vi "Simple_DAQ_PressureTime_Graph.vi"() -> ()   [LabVIEW 2021]
panel:
  in  "See Log FilePath":bool
  out "Log File Name":string
  out "Log Date & Time":string
  out "Log File Path":path
  out "error out":errorcluster
  in  "Start Logging":bool
  out "Pressure Chart":dbl[](graph)
  out "Date & Time":string
  out "Pressure (Bar)":dbl format="%#2_4f"
  in  "Start Aquisition":bool
  out "Voltage Detected":dbl format="%0.2f"
  in  "Stop Button":bool
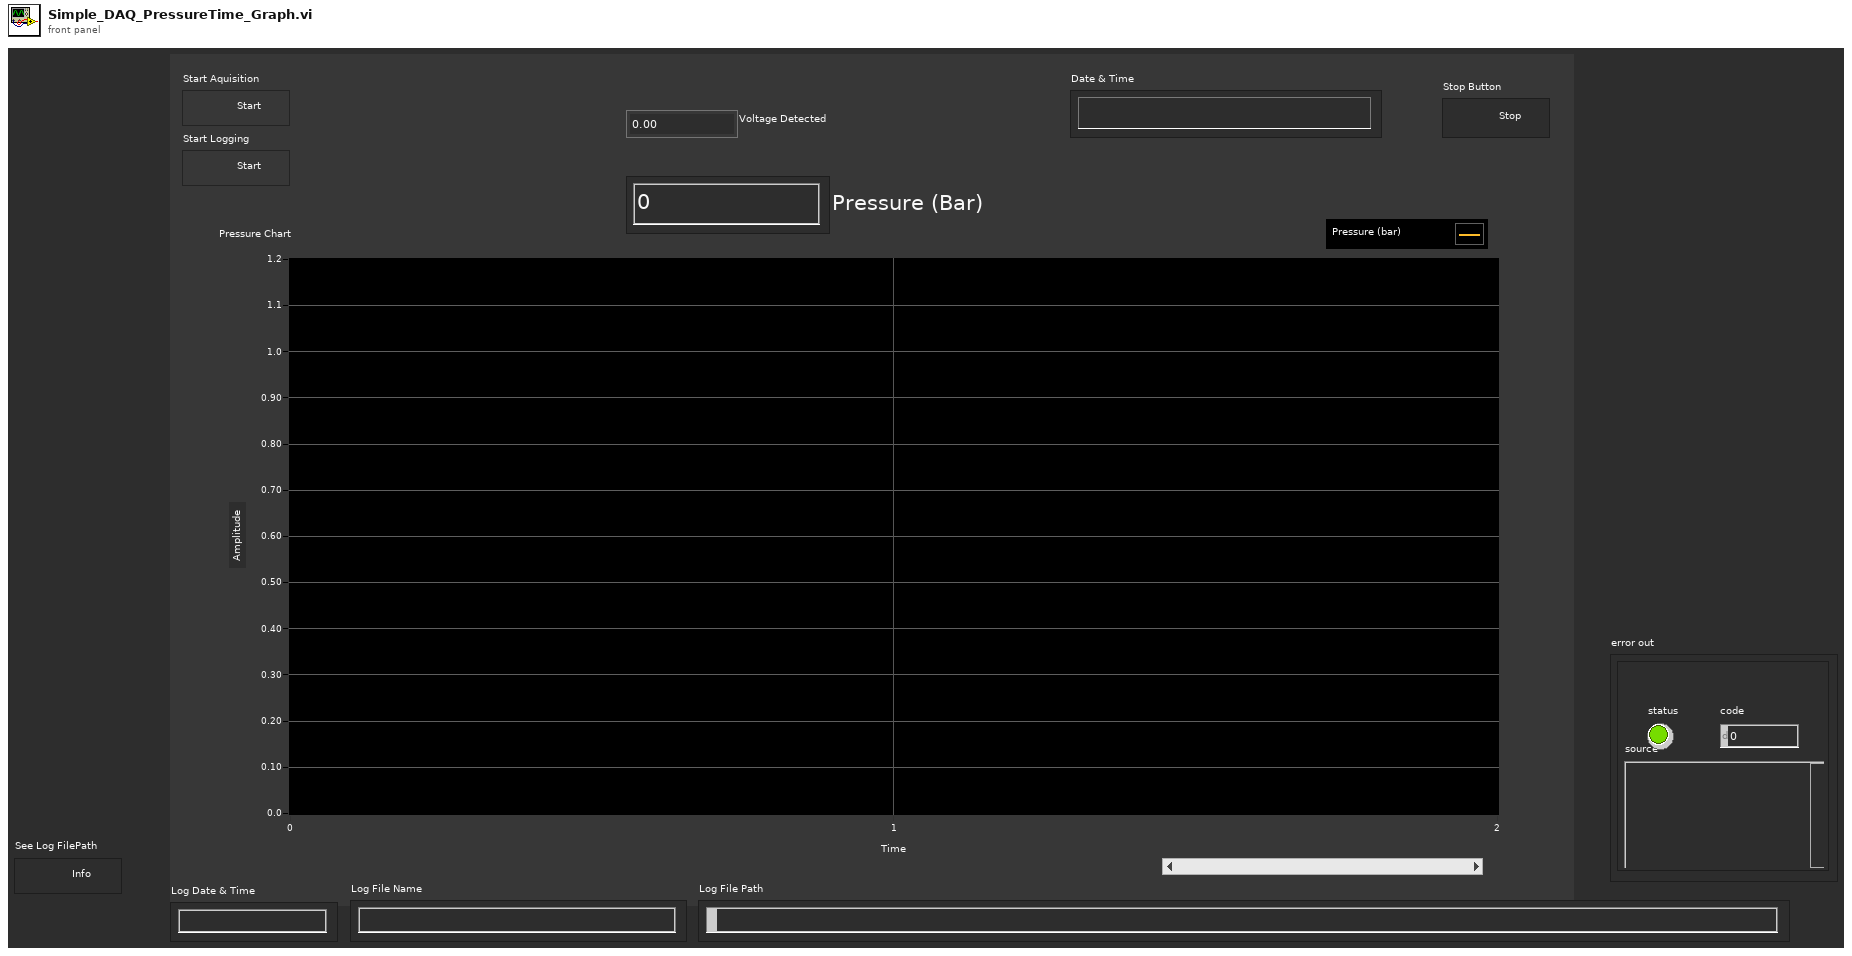
[diagram p1: front panel]
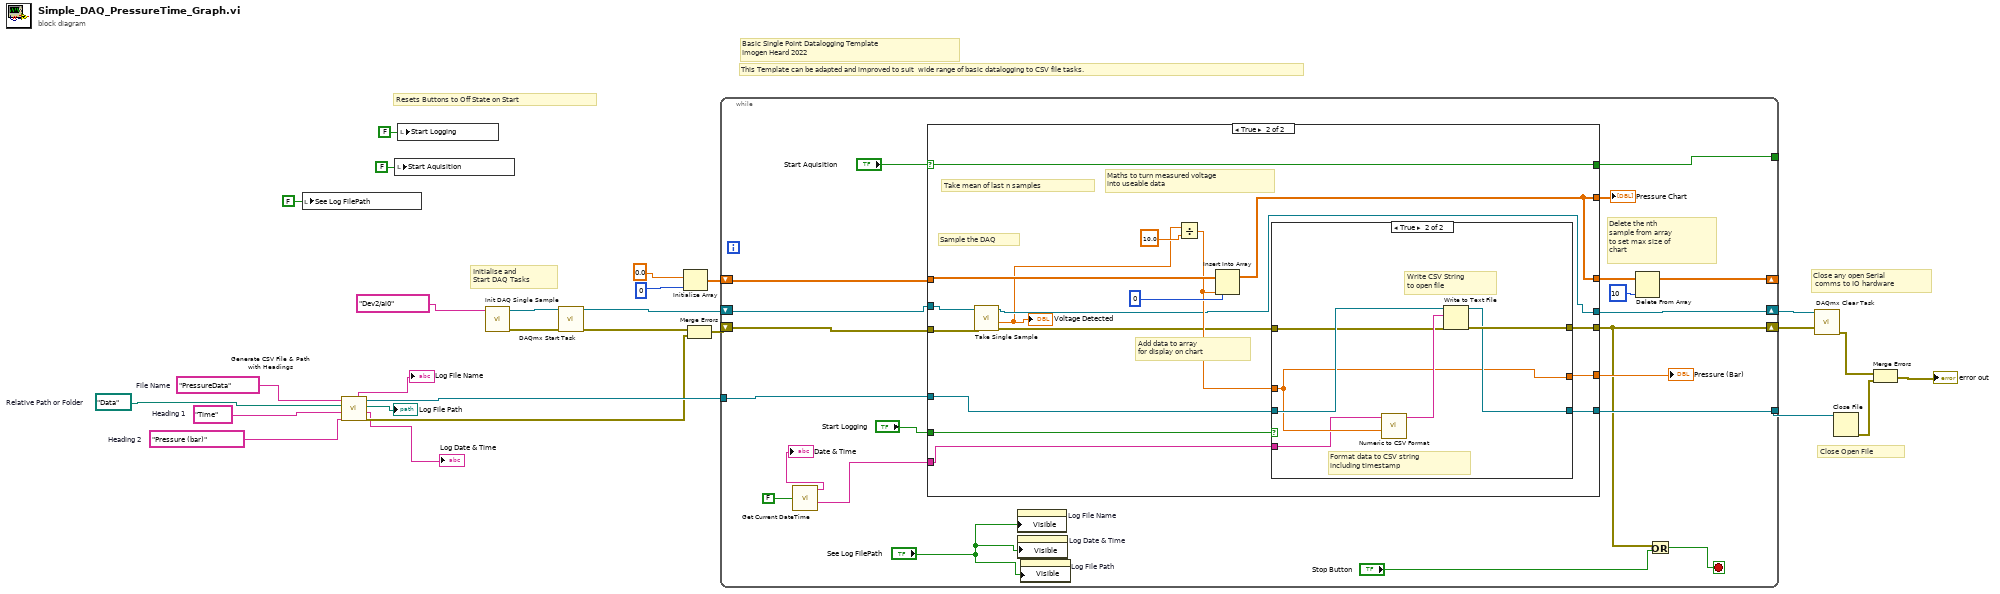
[diagram p0: block diagram]
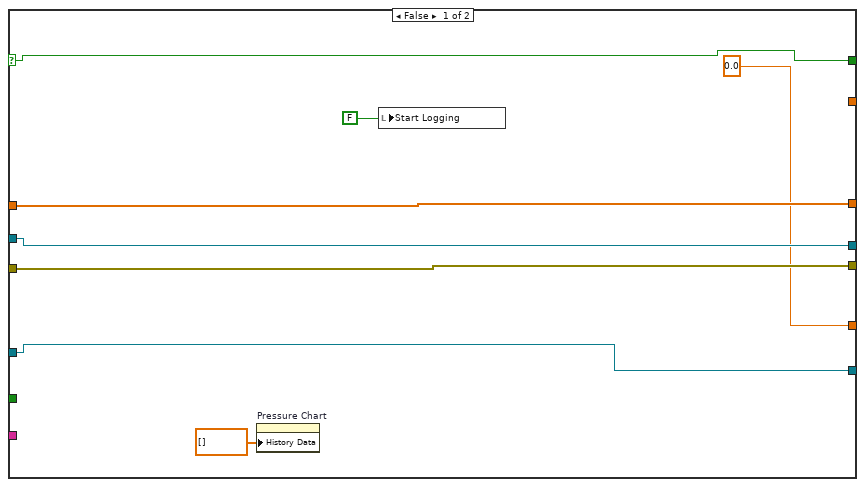
[diagram p2: hidden frame]
diagram:
  w8 = "Time"  # Heading 1
  w4 = "Pressure (bar)"  # Heading 2
  w2 = "PressureData"  # File Name
  w3 = path "Data"  # Relative Path or Folder
  # "Close Open File"
  # "Close any open Serial\n comms to IO hardware"
  # "This Template can be adapted and improved to suit  wide range of basic datalogging to CSV file tasks."
  # "Basic Single Point Datalogging Template\nImogen Heard 2022"
  # "Initialise and \nStart DAQ Tasks"
  # "Resets Buttons to Off State on Start"
  n1 = local write "See Log FilePath"(FALSE ("See Log FilePath")) -> ()
  n2 = call "Generate CSV File & Path with Headings.vi"("Heading 2"=w4, "Heading 1"=w8, "Relative Path or Folder"=w3, "File Name"=w2) -> ("error out"=w14:errorcluster, "Log Date & Time"=→"Log Date & Time":string, "Log File Path"=→"Log File Path":path, "Byte Stream File out"=w15:refnum<file>, "Log File Name"=→"Log File Name":string)  [unwired: 3 in]
  n3 = local write "Start Aquisition"(FALSE ("Start Aquisition")) -> ()
  n4 = local write "Start Logging"(FALSE ("Start Logging")) -> ()
  n5 = call "Init DAQ Single Sample.vi"("physical channels"=tag "Dev2/ai0") -> ("error out"=w19:errorcluster, "Refnum out"=w27:refnum<k21>)  [unwired: 9 in]
  n6 = call <vilib>:"DAQmx Start Task.vi"("task/channels in"=w27, "error in"=w19) -> ("task out"=w26:refnum<k21>, "error out"=w17:errorcluster)  [unwired: 12 in]
  n7 = Initialize Array(0.0 ("y"), 0 ("dimension size")) -> (w23:dbl[])
  n8 = Merge Errors(w17, w14) -> (w18:errorcluster)
  n9 = while {
    shift-right: [w46] -> w25
    shift-left: w26 -> [w48]
    shift-right: [w28] -> w12
    shift-left: w18 -> [w47]
    shift-right: [w41] -> _
    shift-left: w23 -> [w45]
    tunnel: [w39] -> w13
    tunnel: w15 -> [w37]
    tunnel: [w33] -> _
    stop <- w30 stop-if-true
    # "Delete the nth\nsample from array\nto set max size of \nchart"
    n10 = call "Get Current DateTime.vi"("Leading Apostrophe"=FALSE) -> ("Time String"=w36:string, "Date/Time String"=→"Date & Time":string)  [unwired: 7 in, 2 out]
    n11 = case shown="True" "Start Aquisition" {
      selector: "Start Aquisition" -> [w49 w62]
      tunnel: w48 -> [w56 w60]
      tunnel: w47 -> [w55 w61]
      tunnel: [w55 w69] -> w28
      tunnel: [w56 w59] -> w46
      tunnel: w45 -> [w53 w71]
      tunnel: [w53 w70] -> w42
      tunnel: [0.0 w67] -> w40
      tunnel: [_ w70] -> w44
      tunnel: "Start Logging" -> [_ w63]
      tunnel: w37 -> [w51 w66]
      tunnel: [w51 w65] -> w39
      tunnel: w36 -> [_ w64]
      tunnel: [w49 w62] -> w33
      frame False {
        n12 = property on="Pressure Chart" class="WFChart (strict)"("History Data"=dbl[] []) -> ()  [unwired: 2 in, 2 out]
        n13 = local write "Start Logging"(FALSE ("Start Aquisition")) -> ()
      }
      frame True {
        # "Add data to array\nfor display on chart"
        # "Maths to turn measured voltage\ninto useable data"
        # "Take mean of last n samples"
        # "Sample the DAQ"
        n14 = call "Take Single Sample.vi"("error in (no error)"=w61, "Refnum in"=w60) -> ("error out"=w58:errorcluster, "Voltage Detected"=w57:dbl, "Refnum out"=w59:refnum<k21>)  [unwired: 7 in]
        "Voltage Detected" <- w57
        n15 = Divide(x=w57, y=10.0) -> (x/y=w68:dbl)
        n16 = Insert Into Array(array=w71, index=0, new element=w68) -> (w70:dbl[])
        n17 = case shown="True" w63 {
          tunnel: [w74 w82] -> w69
          tunnel: w68 -> [w76 w79]
          tunnel: [w76 w79] -> w67
          tunnel: w66 -> [w75 w83]
          tunnel: [w75 w81] -> w65
          tunnel: w64 -> [_ w78]
          tunnel: w58 -> [w74 w77]
          frame False {
          }
          frame True {
            # "Write CSV String\nto open file"
            # "Format data to CSV string\nincluding timestamp"
            n18 = call "Numeric to CSV Format.vi"("Numeric"=w79, "Time String"=w78) -> ("spreadsheet string"=w80:string)  [unwired: 9 in]
            n19 = Write to Text File(file (use dialog)=w83, text=w80, error in=w77) -> (refnum out=w81:refnum<file>, error out=w82:errorcluster)  [unwired: 1 in, 1 out]
          }
        }
      }
    }
    "Pressure Chart" <- w44
    "Pressure (Bar)" <- w40
    n20 = property on="Log File Name" class="Str"("Visible"="See Log FilePath") -> ()  [unwired: 2 in, 2 out]
    n21 = property on="Log Date & Time" class="Str"("Visible"="See Log FilePath") -> ()  [unwired: 2 in, 2 out]
    n22 = property on="Log File Path" class="Path"("Visible"="See Log FilePath") -> ()  [unwired: 2 in, 2 out]
    n23 = Delete From Array(array=w42, index=10) -> (array with subset deleted=w41:dbl[])  [unwired: 1 in, 1 out]
    n24 = Or(x=w28, y="Stop Button") -> (x .or. y?=w30:bool)
  }
  n25 = call <vilib>:"DAQmx Clear Task.vi"("task in"=w25, "error in"=w12) -> ("error out"=w10:errorcluster)  [unwired: 13 in]
  n26 = Close File(refnum=w13) -> (error out=w9:errorcluster)  [unwired: 1 in, 1 out]
  n27 = Merge Errors(w10, w9) -> (→"error out":errorcluster)
